vi "sbRIO.vi"() -> ()   [LabVIEW 2012]
uses:
  <vilib>/Platform/TimedLoop/XDataNode/timing_clust.ctl
  <vilib>/Platform/TimedLoop/XDataNode/nitl_modes.ctl
  <vilib>/Platform/TimedLoop/XDataNode/wakeup.ctl
  <vilib>/FPGAPlugInAG/sbRIO-9642/niLvFpga_Open_sbRIO-9642.vi
  <vilib>/rvi/interface/common/dynamic/niFpgaDynamicAddResources.vi
  <vilib>/Utility/error.llb/Error Cluster From Error Code.vi
  <vilib>/rvi/errors/niLvFpgaAdjustHostInterfaceError.vi
  <vilib>/FPGAPlugInAG/Dynamic/niLvFpga_Close_Dynamic.vi
  <vilib>/Platform/TimedLoop/XDataNode/XDataNode.xnode
  <vilib>/rvi/interface/nirviOpenFPGA/nirviOpenFPGA.xnode
  FPGA Bitfiles/ReleaseCandidate_FPGATarget_FPGA_LS4xwvBfOfc.lvbitx
  FPGA.vi
  <vilib>/rvi/interface/nirviReadWriteControl/nirviReadWriteControl.xnode
  <vilib>/rvi/interface/nirviCloseFPGA/nirviCloseFPGA.xnode
  NiFpgaLv.dll
  <vilib>/rvi/interface/Simulation/niFpgaSimulationCallBeginRW.vi
  Helper Functions/ProcessorHelperFunctions.lvlib
  <vilib>/Platform/TimedLoop/XDataNode/XDNodeRunTimeDep.lvlib
panel:
  in  "Error Correction Speed":dbl
  out "Wheel Pos/Speed":picture
  out "Simulation Wheel Angles":dbl[](array[numeric])
  in  "Port":u16=2055 min=1025 step=1
  out "RX Data":T1
  in  "stop":bool
  in  "Manual Motor Control":bool=TRUE
  in  "Motor Number":u8
  out "Chassis Temp (C)":dbl
  out "E1":i64
  out "E3":i64
  out "E2":i64
  out "E4":i64
  out "A1":dbl
  out "A3":dbl
  out "A2":dbl
  out "A4":dbl
  out "T1":dbl
  out "T3":dbl
  out "T2":dbl
  out "T4":dbl
  in  "Calibration Mode":bool
  in  "Debug Mode":bool
  out "Wheel Target Angles":dbl[](array[numeric])
  out "Motor Output Values":u16[](array[slide]) scale=0.0..512.0
  in  "Offset1":i64
  in  "Offset3":i64
  in  "Offset2":i64
  in  "Offset4":i64
  # "Manual Motor Control"
  # "Encoder Count Pre Offset"
  # "Override All"
  # "Automatic\n  Control"
  # "Actual Wheel Angles"
  # "Target Wheel Angles"
  # "Wheel Calibration offsets"
  # "Debug"
  # "(ECS models physical \nparamaters of the robot)"
  # "Normal Operation"
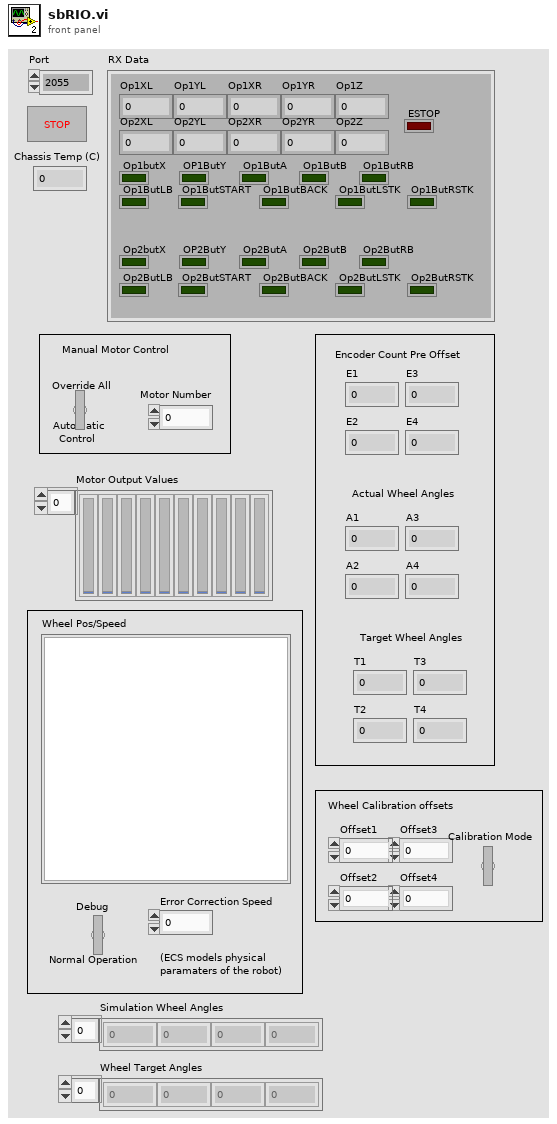
[diagram p1: front panel]
types:
  T1 = cluster{"Op2ButLSTK":bool, "Op2ButRSTK":bool, "Op1ButLSTK":bool, "Op1ButRSTK":bool, "Op1XL":i32, "Op1YL":i32, "Op1XR":i32, "Op1YR":i32, "Op1Z":i32, "Op2XL":i32, "Op2YL":i32, "Op2XR":i32, "Op2YR":i32, "Op2Z":i32, "ESTOP":bool, "Op1butX":bool, "OP1ButY":bool, "Op1ButA":bool, "Op1ButB":bool, "Op1ButRB":bool, "Op1ButLB":bool, "Op2butX":bool, "OP2ButY":bool, "Op2ButA":bool, "Op2ButB":bool, "Op2ButRB":bool, "Op2ButLB":bool, "Op2ButSTART":bool, "Op2ButBACK":bool, "Op1ButSTART":bool, "Op1ButBACK":bool}
  T2 = typedef "XDNodeRunTimeDep.lvlib/timing_clust.ctl" = cluster{"Expected End [f-1]":u64, "Actual End [f-1]":u64, "Finished Late? [f-1]":bool, "Expected End [i-1]":u64, "Actual End [i-1]":u64, "Finished Late? [i-1]":bool, "Expected Start [i]":u64, "Actual Start [i]":u64, "Expected Start [f]":u64, "Actual Start [f]":u64, "Source Name":string, "Structure Name":string, "Period":i64, "Deadline":i64, "Offset":i64, "Start":i64, "Priority":i32, "Timeout":i32, "Mode":T3, "Wakeup Reason":T4, "Error":errorcluster, "Source Type":string, "Secondary Source Type":string, "Global End Time":u64, "Global Start Time":u64, "Frame Duration":u64, "Iteration Duration":u64, "Assigned CPU":i32, "I/O Scan Engine Mode":u32}
  T3 = typedef "XDNodeRunTimeDep.lvlib/nitl_modes.ctl" = enum32{"No Change", "Process missed periods, maintain original phase", "Discard missed periods, maintain original phase", "Process missed periods, ignore original phase", "Discard missed periods, ignore original phase"}
  T4 = typedef "XDNodeRunTimeDep.lvlib/wakeup.ctl" = enum32{"Normal", "Aborted", "Asynchronous wakeup", "Timing source error", "Timed loop error", "Timeout"}
  T5 = cluster{"Target Angles[0]":dbl, "Target Angles[1]":dbl, "Target Angles[2]":dbl, "Target Angles[3]":dbl}
  T6 = cluster{"MotorsOut[0]":u16, "MotorsOut[1]":u16, "MotorsOut[2]":u16, "MotorsOut[3]":u16, "MotorsOut[4]":u16, "MotorsOut[5]":u16, "MotorsOut[6]":u16, "MotorsOut[7]":u16, "MotorsOut[8]":u16, "MotorsOut[9]":u16, "MotorsOut[10]":u16, "MotorsOut[11]":u16}
  T7 = cluster{"[0]":dbl, "[1]":dbl, "[2]":dbl, "[3]":dbl, "[4]":dbl, "[5]":dbl, "[6]":dbl, "[7]":dbl, "[8]":dbl}
  T8 = cluster{"[0]":u16, "[1]":u16, "[2]":u16, "[3]":u16}
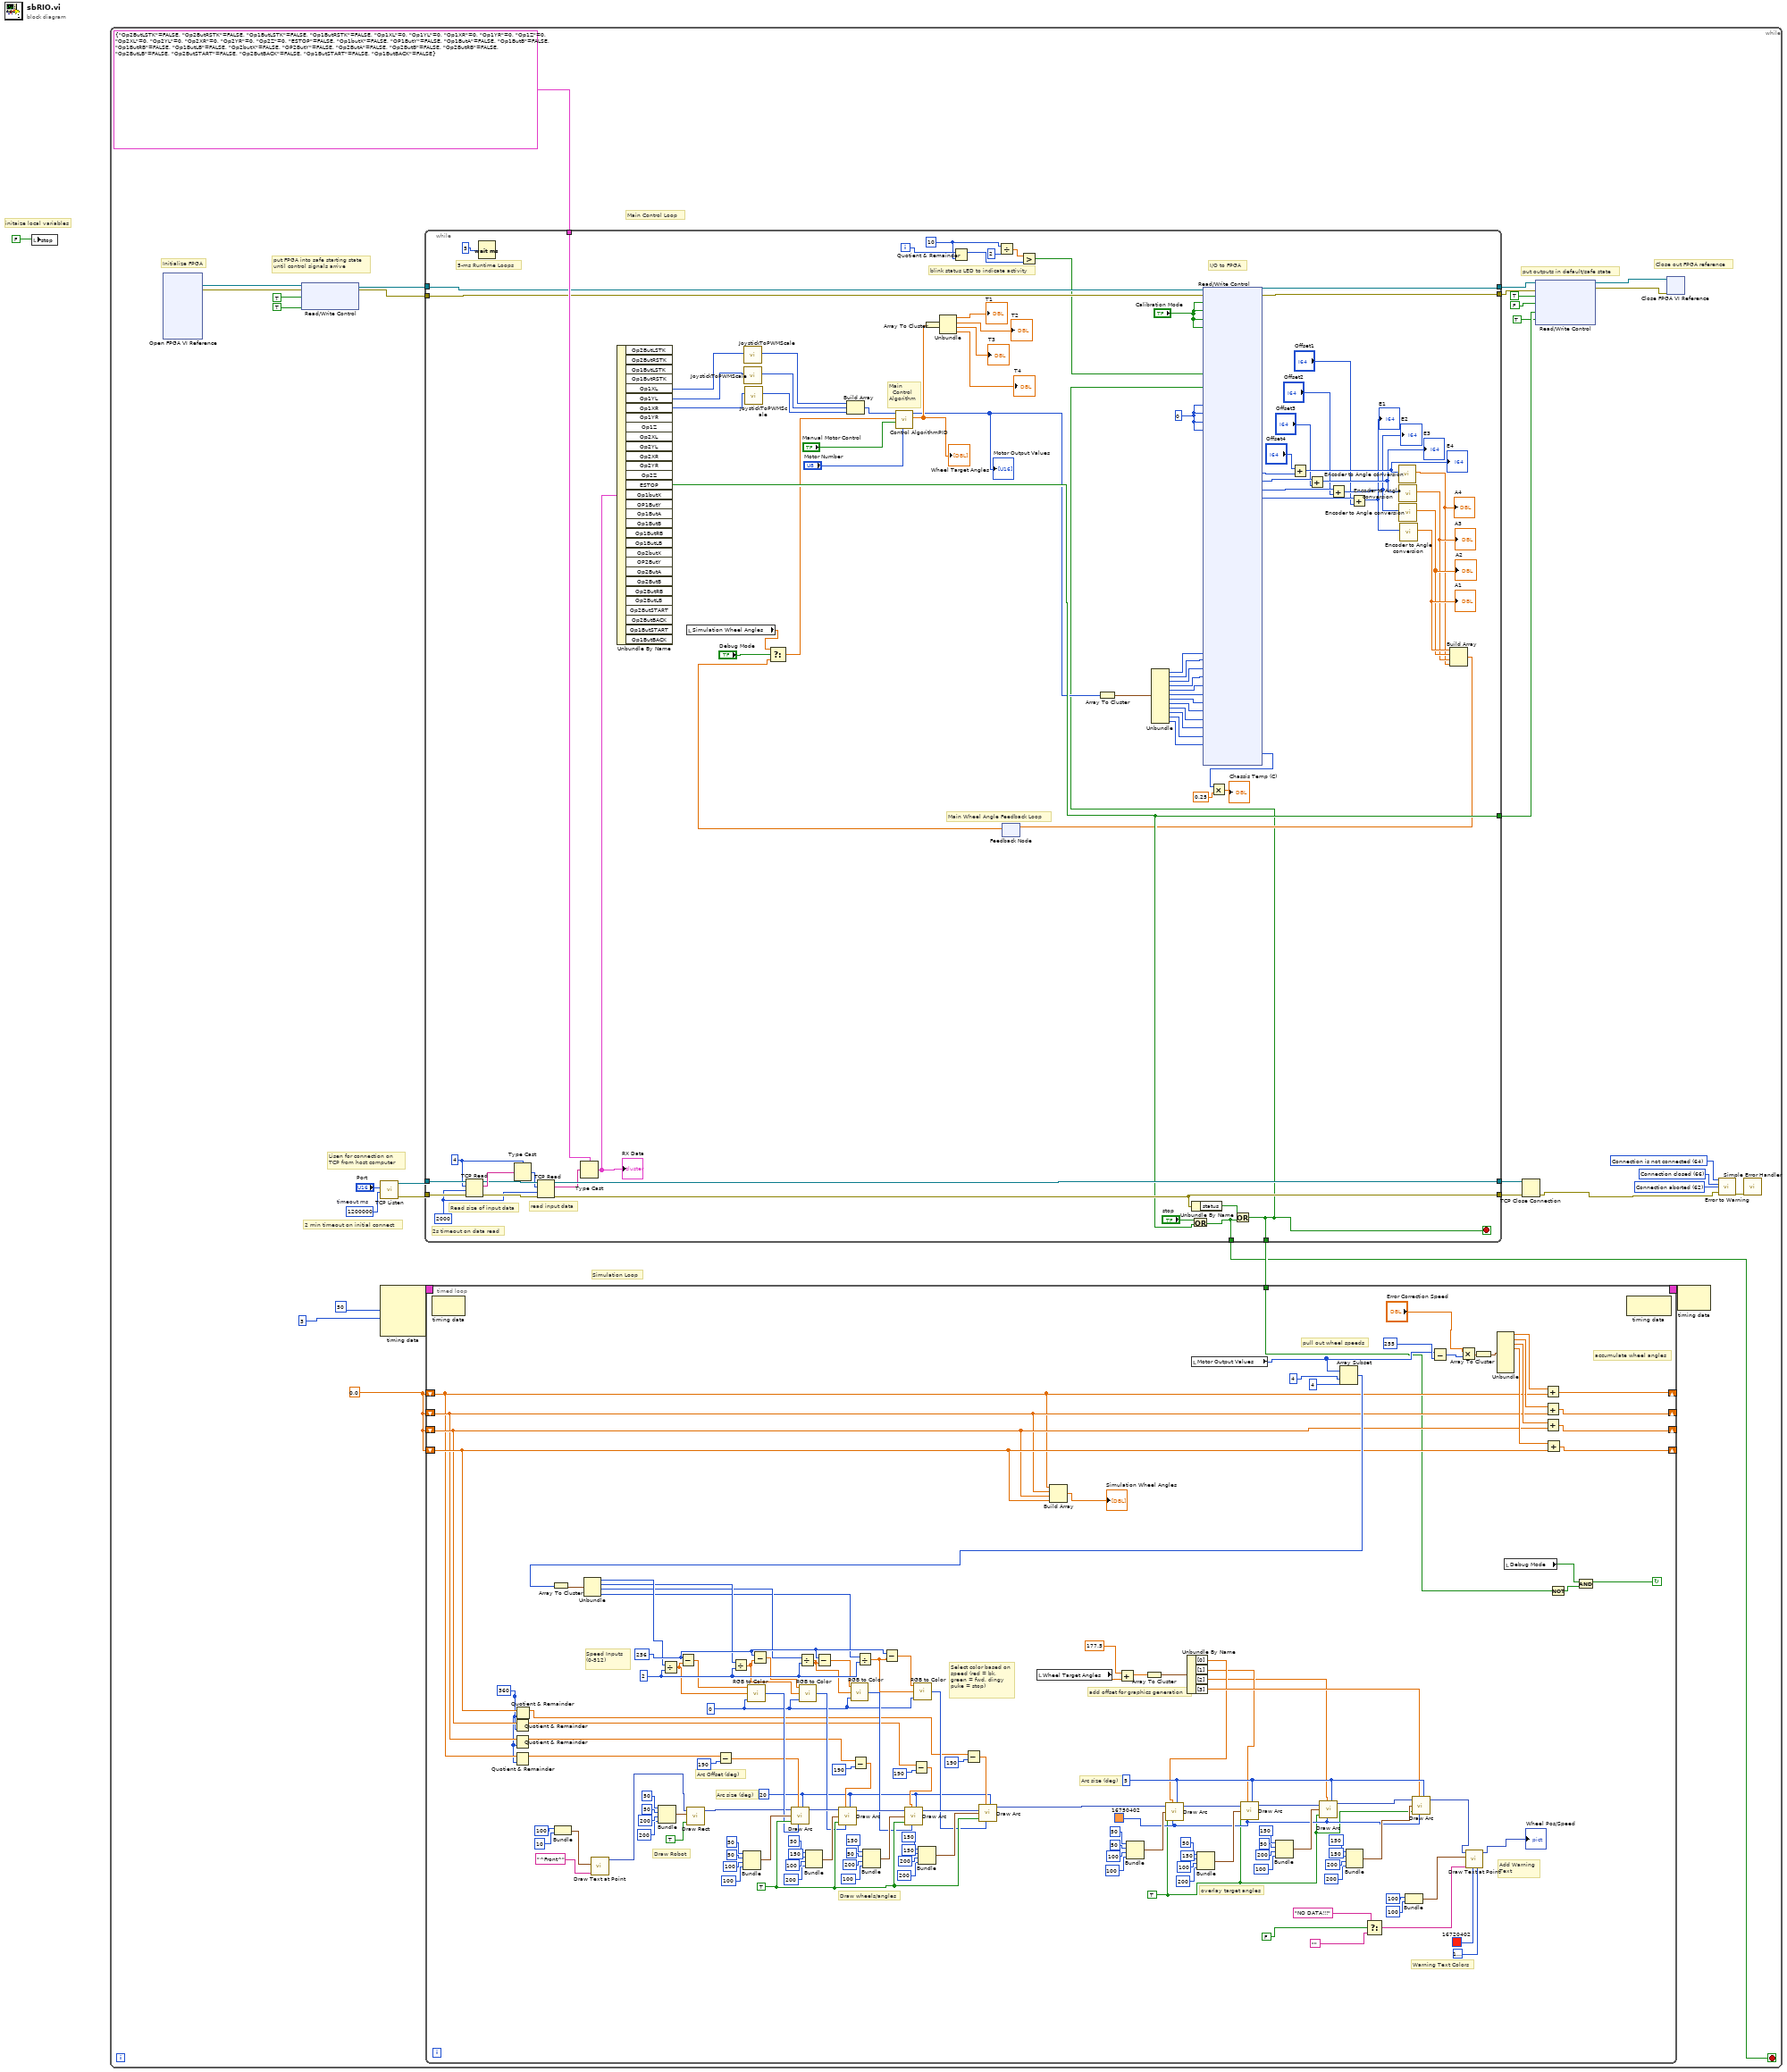
[diagram p0: block diagram]
diagram:
  # "initaize local variables"
  n1 = local write "stop"(FALSE) -> ()
  n2 = while {
    stop <- w2 stop-if-true
    w5 = 0.0
    w25 = 1200000  # timeout ms
    w29 = 62 items=["No Error", "Argument Error", "Memory Full", "Out of Zone", "End of File", "File Already Open", "Generic File IO Error", "File Not Found", "File Permission Error", "Disk Full", "Duplicate Path", "Too Many Files Open", "Not Enabled", "Resource File Not Found", "Cannot Add Resource", "Resource Not Found", "Image Not Found", "Image Memory Error", "Pen Does Not Exist", "Config Bad Type", "Config Token Not Found", "Config Parse Error", "Config Memory Error", "Bad External Code Format", "Bad External Code Offset", "External Code Not Present", "Null Window", "Destroy Window Mixup", "Null Menu", "Print Aborted", "Bad Print Record", "Print Driver Error", "Windows Error During Print", "Memory Error During Print", "Print Dialog Error", "Generic Print Error", "Invalid Device Refnum", "Device Not Found", "Device Parameter Error", "Device Unit Error", "Can't Open Device", "Device Call Aborted", "Generic Error", "Cancelled By User", "Object ID Too Low", "Object ID Too High", "Object Not In Heap", "Unknown Heap", "Bad DefProc ID", "DefProc Not In Table", "Message Out Of Range", "Null Method", "Unknown Message", "Manager Call Not Supported", "Bad address", "Connection In progress", "Connection timed out", "Connection is already in progress", "Network attribute not supported", "Network error", "Address in use", "System out of memory", "Connection aborted", "Connection refused", "Connection is not connected", "Connection is already connected", "Connection closed", "Initialize error (interapplication manager)", "Bad occurrence", "Wait on unbound occurrence handler", "Occurrence queue overflow", "Bad path", "Semaphore not signaled", "Unrecognized type (interapplication manager)"] ("1st Error to Convert")
    w30 = 66 items=["No Error", "Argument Error", "Memory Full", "Out of Zone", "End of File", "File Already Open", "Generic File IO Error", "File Not Found", "File Permission Error", "Disk Full", "Duplicate Path", "Too Many Files Open", "Not Enabled", "Resource File Not Found", "Cannot Add Resource", "Resource Not Found", "Image Not Found", "Image Memory Error", "Pen Does Not Exist", "Config Bad Type", "Config Token Not Found", "Config Parse Error", "Config Memory Error", "Bad External Code Format", "Bad External Code Offset", "External Code Not Present", "Null Window", "Destroy Window Mixup", "Null Menu", "Print Aborted", "Bad Print Record", "Print Driver Error", "Windows Error During Print", "Memory Error During Print", "Print Dialog Error", "Generic Print Error", "Invalid Device Refnum", "Device Not Found", "Device Parameter Error", "Device Unit Error", "Can't Open Device", "Device Call Aborted", "Generic Error", "Cancelled By User", "Object ID Too Low", "Object ID Too High", "Object Not In Heap", "Unknown Heap", "Bad DefProc ID", "DefProc Not In Table", "Message Out Of Range", "Null Method", "Unknown Message", "Manager Call Not Supported", "Bad address", "Connection In progress", "Connection timed out", "Connection is already in progress", "Network attribute not supported", "Network error", "Address in use", "System out of memory", "Connection aborted", "Connection refused", "Connection is not connected", "Connection is already connected", "Connection closed", "Initialize error (interapplication manager)", "Bad occurrence", "Wait on unbound occurrence handler", "Occurrence queue overflow", "Bad path", "Semaphore not signaled", "Unrecognized type (interapplication manager)"] ("1st Error to Convert")
    w31 = 64 items=["No Error", "Argument Error", "Memory Full", "Out of Zone", "End of File", "File Already Open", "Generic File IO Error", "File Not Found", "File Permission Error", "Disk Full", "Duplicate Path", "Too Many Files Open", "Not Enabled", "Resource File Not Found", "Cannot Add Resource", "Resource Not Found", "Image Not Found", "Image Memory Error", "Pen Does Not Exist", "Config Bad Type", "Config Token Not Found", "Config Parse Error", "Config Memory Error", "Bad External Code Format", "Bad External Code Offset", "External Code Not Present", "Null Window", "Destroy Window Mixup", "Null Menu", "Print Aborted", "Bad Print Record", "Print Driver Error", "Windows Error During Print", "Memory Error During Print", "Print Dialog Error", "Generic Print Error", "Invalid Device Refnum", "Device Not Found", "Device Parameter Error", "Device Unit Error", "Can't Open Device", "Device Call Aborted", "Generic Error", "Cancelled By User", "Object ID Too Low", "Object ID Too High", "Object Not In Heap", "Unknown Heap", "Bad DefProc ID", "DefProc Not In Table", "Message Out Of Range", "Null Method", "Unknown Message", "Manager Call Not Supported", "Bad address", "Connection In progress", "Connection timed out", "Connection is already in progress", "Network attribute not supported", "Network error", "Address in use", "System out of memory", "Connection aborted", "Connection refused", "Connection is not connected", "Connection is already connected", "Connection closed", "Initialize error (interapplication manager)", "Bad occurrence", "Wait on unbound occurrence handler", "Occurrence queue overflow", "Bad path", "Semaphore not signaled", "Unrecognized type (interapplication manager)"] ("1st Error to Convert")
    # "Simulation Loop"
    # "Main Control Loop"
    # "put FPGA into safe starting state\nuntil control signals arrive"
    # "put outputs in default/safe state"
    # "Close out FPGA reference"
    # "Initialize FPGA"
    # "2 min timeout on initial connect"
    # "Lisen for connection on \nTCP from host computer"
    n3 = xnode "Open FPGA VI Reference"() -> ("FPGA VI Reference Out"=w16:refnum<k20>, "error out"=w15:errorcluster)  [unwired: 2 in]
    n4 = xnode "Read/Write Control"("FPGA VI Reference In"=w16, "error in"=w15, "Stop All Motors"=TRUE, "Status LED"=TRUE) -> ("FPGA VI Reference Out"=w14:refnum<k20>, "error out"=w13:errorcluster)
    n5 = call <vilib>:"TCP Listen.vi"("timeout ms (wait forever: -1)"=w25, "port"="Port") -> ("error out"=w23:errorcluster, "connection ID"=w24:refnum<k5>)  [unwired: 5 in, 3 out]
    n6 = node-c288(50, 3) -> (w34:T2)  [unwired: 2 in]
    n7 = while {
      tunnel: w23 -> [w261]
      tunnel: w24 -> [w262]
      tunnel: [w263] -> w22
      tunnel: [w258] -> w21
      tunnel: T1 {"Op2ButLSTK"=FALSE, "Op2ButRSTK"=FALSE, "Op1ButLSTK"=FALSE, "Op1ButRSTK"=FALSE, "Op1XL"=0, "Op1YL"=0, "Op1XR"=0, "Op1YR"=0, "Op1Z"=0, "Op2XL"=0, "Op2YL"=0, "Op2XR"=0, "Op2YR"=0, "Op2Z"=0, "ESTOP"=FALSE, "Op1butX"=FALSE, "OP1ButY"=FALSE, "Op1ButA"=FALSE, "Op1ButB"=FALSE, "Op1ButRB"=FALSE, "Op1ButLB"=FALSE, "Op2butX"=FALSE, "OP2ButY"=FALSE, "Op2ButA"=FALSE, "Op2ButB"=FALSE, "Op2ButRB"=FALSE, "Op2ButLB"=FALSE, "Op2ButSTART"=FALSE, "Op2ButBACK"=FALSE, "Op1ButSTART"=FALSE, "Op1ButBACK"=FALSE} -> [w255]
      tunnel: w14 -> [w251]
      tunnel: w13 -> [w250]
      tunnel: [w249] -> w20
      tunnel: [w248] -> w19
      tunnel: [w241] -> w8
      tunnel: [w193] -> w3
      tunnel: [w184] -> w2
      i -> [w247]
      stop <- w193 stop-if-true
      w208 = 0
      w243 = 10
      w254 = 2000
      w259 = 4
      # "Main\n  Control\nAlgorithm"
      # "Main Wheel Angle Feedback Loop"
      # "blink status LED to indicate activity"
      # "I/O to FPGA"
      # "2s timeout on data read"
      # "read input data"
      # "Read size of input data"
      # "5-ms Runtime Loops"
      n8 = TCP Read(connection ID=w262, bytes to read=w259, error in (no error)=w261, 9:w254) -> (connection ID out=w266:refnum<k5>, data out=w267:string, error out=w265:errorcluster)  [unwired: 1 in]
      n9 = Wait (ms)(milliseconds to wait=u32 5) -> ()  [unwired: 1 out]
      n10 = Type Cast(type=w259, x=w267) -> (*(type *) &x=w264:i32)
      n11 = TCP Read(connection ID=w266, bytes to read=w264, error in (no error)=w265, 9:w254) -> (connection ID out=w263:refnum<k5>, data out=w260:string, error out=w258:errorcluster)  [unwired: 1 in]
      n12 = Type Cast(type=w255, x=w260) -> (*(type *) &x=w253:T1)
      "RX Data" <- w253
      n13 = Unbundle By Name(w253) -> ("Op1XL"=w206:i32, "Op1YL"=w205:i32, "Op1XR"=w204:i32, "ESTOP"=w241:bool)  [unwired: 27 out]
      n14 = local read "Simulation Wheel Angles"() -> (w198:dbl[])
      n15 = call "JoystickToPWMScale.vi"("Numeric"=w206) -> ("Numeric 2"=w203:u16)  [unwired: 10 in]
      n16 = call "JoystickToPWMScale.vi"("Numeric"=w205) -> ("Numeric 2"=w202:u16)  [unwired: 10 in]
      n17 = call "JoystickToPWMScale.vi"("Numeric"=w204) -> ("Numeric 2"=w201:u16)  [unwired: 10 in]
      n18 = Build Array(w203, w202, w201) -> (w207:u16[])
      n19 = Quotient & Remainder(x=w247, y=w243) -> (x-y*floor(x/y)=w245:i32)  [unwired: 1 out]
      n20 = Divide(x=w243, y=2) -> (x/y=w244:dbl)
      n21 = feedback #1() -> (w199:dbl[])  [unwired: 1 in]
      n22 = Select(t=w198, s="Debug Mode", f=w199) -> (s? t:f=w196:dbl[])
      n23 = call "Control AlgorithmPID.vi"("Motor to Control"="Motor Number", "Manual Control"="Manual Motor Control", "Angles In"=w196, "JoystickIn"=w207) -> ("Target Angles"=w195:dbl[], "MotorsOut"=w194:u16[])  [unwired: 5 in]
      "Wheel Target Angles" <- w195
      "Motor Output Values" <- w194
      n24 = Array To Cluster(array=w195) -> (cluster=w223:T5)
      n25 = Unbundle(w223) -> ("Target Angles[0]"=→"T1":dbl, "Target Angles[1]"=→"T2":dbl, "Target Angles[2]"=→"T3":dbl, "Target Angles[3]"=→"T4":dbl)
      n26 = Greater?(x=w244, y=w245) -> (0:w242:bool)
      n27 = Array To Cluster(array=w194) -> (cluster=w229:T6)
      n28 = Unbundle(w229) -> ("MotorsOut[0]"=w239:u16, "MotorsOut[1]"=w238:u16, "MotorsOut[2]"=w237:u16, "MotorsOut[3]"=w236:u16, "MotorsOut[4]"=w235:u16, "MotorsOut[5]"=w234:u16, "MotorsOut[6]"=w233:u16, "MotorsOut[7]"=w232:u16, "MotorsOut[8]"=w231:u16, "MotorsOut[9]"=w230:u16, "MotorsOut[10]"=w228:u16, "MotorsOut[11]"=w227:u16)
      n29 = Unbundle By Name(w258) -> ("status"=w257:bool)
      n30 = Or(x="stop", y=w241) -> (x .or. y?=w184:bool)
      n31 = Or(x=w257, y=w184) -> (x .or. y?=w193:bool)
      n32 = xnode "Read/Write Control"("FPGA VI Reference In"=w251, "error in"=w250, "Cal. 4"="Calibration Mode", "Cal. 3"="Calibration Mode", "Cal.2"="Calibration Mode", "Cal.1"="Calibration Mode", "Status LED"=w242, "Stop All Motors"=w193, "Analog 3"=w208, "Analog 1"=w208, "Analog 4"=w208, "Analog 2"=w208, "Motor1"=w239, "Motor2"=w238, "Motor3"=w237, "Motor4"=w236, "Motor5"=w235, "Motor6"=w234, "Motor7"=w233, "Motor8"=w232, "Motor9"=w231, "Motor10"=w230, "Motor11"=w228, "Motor12"=w227) -> ("FPGA VI Reference Out"=w249:refnum<k20>, "error out"=w248:errorcluster, "Encoder4"=w218:i64, "Encoder3"=w217:i64, "Encoder2"=w216:i64, "Encoder1"=w215:i64, "Chasis Temp"=w224:i16)  [unwired: 15 in, 13 out]
      n33 = Multiply(x=w224, y=0.25) -> (x*y=→"Chassis Temp (C)":dbl)
      n34 = Add(x="Offset4", y=w218) -> (x+y=w192:i64)
      "E4" <- w192
      n35 = Add(x=w217, y="Offset3") -> (x+y=w190:i64)
      "E3" <- w190
      n36 = Add(x=w216, y="Offset2") -> (x+y=w189:i64)
      "E2" <- w189
      n37 = Add(x=w215, y="Offset1") -> (x+y=w188:i64)
      "E1" <- w188
      n38 = call "Encoder to Angle conversion.vi"("Input"=w192) -> ("Output"=w211:dbl)  [unwired: 10 in]
      "A4" <- w211
      n39 = call "Encoder to Angle conversion.vi"("Input"=w190) -> ("Output"=w212:dbl)  [unwired: 10 in]
      "A3" <- w212
      n40 = call "Encoder to Angle conversion.vi"("Input"=w189) -> ("Output"=w213:dbl)  [unwired: 10 in]
      "A2" <- w213
      n41 = call "Encoder to Angle conversion.vi"("Input"=w188) -> ("Output"=w214:dbl)  [unwired: 10 in]
      "A1" <- w214
      n42 = Build Array(w214, w213, w212, w211) -> (w210:dbl[])
      n43 = feedback-in #1(w210) -> ()
    }
    n44 = timed-loop {
      timing: w34 -> [_]
      timing-out: [_] -> w33
      shift-right: [w171] -> _
      shift-left: w5 -> [w43]
      shift-right: [w170] -> _
      shift-left: w5 -> [w45]
      shift-right: [w172] -> _
      shift-left: w5 -> [w41]
      shift-right: [w173] -> _
      shift-left: w5 -> [w39]
      tunnel: w3 -> [w35]
      stop <- w37 continue-if-true
      w38 = 360
      w65 = TRUE
      w68 = 5
      w69 = u32 16750402
      w109 = 20
      w111 = 0
      w127 = 2
      w128 = 256
      w140 = TRUE
      # "add offset for graphics generation"
      # "pull out wheel speeds"
      # "Arc size (deg)"
      # "overlay target angles"
      # "Add Warning\nText"
      # "Warning Text Colors"
      # "Arc Offset (deg)"
      # "Arc size (deg)"
      # "Speed Inputs (0-512)"
      # "Draw wheels/angles"
      # "Select color based on speed (red = bk, green = fwd, dingy puke = stop)"
      # "Draw Robot"
      # "accumulate wheel angles"
      n45 = node-c288() -> ()  [unwired: 1 in, 1 out]
      n46 = Quotient & Remainder(x=w43, y=w38) -> (x-y*floor(x/y)=w44:dbl)  [unwired: 1 out]
      n47 = Quotient & Remainder(x=w41, y=w38) -> (x-y*floor(x/y)=w42:dbl)  [unwired: 1 out]
      n48 = Quotient & Remainder(x=w39, y=w38) -> (x-y*floor(x/y)=w40:dbl)  [unwired: 1 out]
      n49 = Quotient & Remainder(x=w45, y=w38) -> (x-y*floor(x/y)=w46:dbl)  [unwired: 1 out]
      n50 = Bundle(100, 10) -> (w104:cluster{i32, i32})  [unwired: 1 in]
      n51 = call <vilib>:"Draw Text at Point.vi"("text"="^Front^", "origin"=w104) -> ("new picture"=w108:picture)  [unwired: 8 in, 1 out]
      n52 = Bundle(50, 50, 200, 200) -> (w131:cluster{i32, i32, i32, i32})  [unwired: 1 in]
      n53 = call <vilib>:"Draw Rect.vi"("picture"=w108, "rect"=w131, "fill?(F)"=TRUE) -> ("new picture"=w129:picture)  [unwired: 6 in]
      n54 = Subtract(x=w40, y=190) -> (x-y=w117:dbl)
      n55 = Bundle(50, 50, 100, 100) -> (w157:cluster{i32, i32, i32, i32})  [unwired: 1 in]
      n56 = Bundle(50, 150, 100, 200) -> (w143:cluster{i32, i32, i32, i32})  [unwired: 1 in]
      n57 = Subtract(x=w42, y=190) -> (x-y=w113:dbl)
      n58 = Bundle(150, 50, 200, 100) -> (w142:cluster{i32, i32, i32, i32})  [unwired: 1 in]
      n59 = Subtract(x=w44, y=190) -> (x-y=w112:dbl)
      n60 = Bundle(150, 150, 200, 200) -> (w141:cluster{i32, i32, i32, i32})  [unwired: 1 in]
      n61 = Subtract(x=w46, y=190) -> (x-y=w110:dbl)
      n62 = local read "Wheel Target Angles"() -> (w54:dbl[])
      n63 = Build Array(w39, w41, w43, w45) -> (→"Simulation Wheel Angles":dbl[])
      n64 = Add(x=177.5, y=w54) -> (x+y=w51:dbl[])
      n65 = Bundle(50, 50, 100, 100) -> (w87:cluster{i32, i32, i32, i32})  [unwired: 1 in]
      n66 = Array To Cluster(array=w51) -> (cluster=w67:T7)
      n67 = Unbundle By Name(w67) -> ("[0]"=w49:dbl, "[1]"=w48:dbl, "[2]"=w47:dbl, "[3]"=w66:dbl)
      n68 = local read "Motor Output Values"() -> (w55:u16[])
      n69 = Bundle(50, 150, 100, 200) -> (w81:cluster{i32, i32, i32, i32})  [unwired: 1 in]
      n70 = Bundle(150, 50, 200, 100) -> (w76:cluster{i32, i32, i32, i32})  [unwired: 1 in]
      n71 = Array Subset(array=w55, index=4, length=4) -> (w60:u16[])
      n72 = Array To Cluster(array=w60) -> (cluster=w61:T8)
      n73 = Unbundle(w61) -> ("[0]"=w59:u16, "[1]"=w58:u16, "[2]"=w57:u16, "[3]"=w56:u16)
      n74 = Divide(x=w59, y=w127) -> (x/y=w126:dbl)
      n75 = Subtract(x=w128, y=w126) -> (x-y=w123:dbl)
      n76 = Divide(x=w58, y=w127) -> (x/y=w125:dbl)
      n77 = call <vilib>:"RGB to Color.vi"("B"=w111, "G"=w126, "R"=w123) -> ("Color"=w139:u32)
      n78 = Subtract(x=w128, y=w125) -> (x-y=w122:dbl)
      n79 = call <vilib>:"Draw Arc.vi"("picture"=w129, "start angle[degrees]"=w117, "rect"=w157, "fill?(F)"=w140, "color(black)"=w139, "arc size[degrees]"=w109) -> ("new picture"=w163:picture)  [unwired: 3 in]
      n80 = Divide(x=w57, y=w127) -> (x/y=w121:dbl)
      n81 = call <vilib>:"RGB to Color.vi"("B"=w111, "G"=w125, "R"=w122) -> ("Color"=w138:u32)
      n82 = Subtract(x=w128, y=w121) -> (x-y=w120:dbl)
      n83 = call <vilib>:"Draw Arc.vi"("picture"=w163, "start angle[degrees]"=w113, "rect"=w143, "fill?(F)"=w140, "color(black)"=w138, "arc size[degrees]"=w109) -> ("new picture"=w162:picture)  [unwired: 3 in]
      n84 = call <vilib>:"RGB to Color.vi"("B"=w111, "G"=w121, "R"=w120) -> ("Color"=w137:u32)
      n85 = Divide(x=w56, y=w127) -> (x/y=w124:dbl)
      n86 = Subtract(x=w128, y=w124) -> (x-y=w119:dbl)
      n87 = call <vilib>:"Draw Arc.vi"("picture"=w162, "start angle[degrees]"=w112, "rect"=w142, "fill?(F)"=w140, "color(black)"=w137, "arc size[degrees]"=w109) -> ("new picture"=w161:picture)  [unwired: 3 in]
      n88 = call <vilib>:"RGB to Color.vi"("B"=w111, "G"=w124, "R"=w119) -> ("Color"=w136:u32)
      n89 = call <vilib>:"Draw Arc.vi"("picture"=w161, "start angle[degrees]"=w110, "rect"=w141, "fill?(F)"=w140, "color(black)"=w136, "arc size[degrees]"=w109) -> ("new picture"=w93:picture)  [unwired: 3 in]
      n90 = call <vilib>:"Draw Arc.vi"("picture"=w93, "start angle[degrees]"=w49, "rect"=w87, "fill?(F)"=w65, "color(black)"=w69, "arc size[degrees]"=w68) -> ("new picture"=w92:picture)  [unwired: 3 in]
      n91 = call <vilib>:"Draw Arc.vi"("picture"=w92, "start angle[degrees]"=w48, "rect"=w81, "fill?(F)"=w65, "color(black)"=w69, "arc size[degrees]"=w68) -> ("new picture"=w75:picture)  [unwired: 3 in]
      n92 = call <vilib>:"Draw Arc.vi"("picture"=w75, "start angle[degrees]"=w47, "rect"=w76, "fill?(F)"=w65, "color(black)"=w69, "arc size[degrees]"=w68) -> ("new picture"=w91:picture)  [unwired: 3 in]
      n93 = Bundle(150, 150, 200, 200) -> (w70:cluster{i32, i32, i32, i32})  [unwired: 1 in]
      n94 = Select(t="NO DATA!!!", s=FALSE, f="") -> (s? t:f=w97:string)
      n95 = Bundle(100, 100) -> (w100:cluster{i32, i32})  [unwired: 1 in]
      n96 = call <vilib>:"Draw Arc.vi"("picture"=w91, "start angle[degrees]"=w66, "rect"=w70, "fill?(F)"=w65, "color(black)"=w69, "arc size[degrees]"=w68) -> ("new picture"=w94:picture)  [unwired: 3 in]
      n97 = Subtract(x=w55, y=255) -> (x-y=w175:i32[])
      n98 = Multiply(x="Error Correction Speed", y=w175) -> (x*y=w169:dbl[])
      n99 = call <vilib>:"Draw Text at Point.vi"("BG color(transparent)"=u32 16777216, "text color(black)"=u32 16720402, "text"=w97, "origin"=w100, "picture"=w94) -> ("new picture"=→"Wheel Pos/Speed":picture)  [unwired: 5 in, 1 out]
      n100 = Array To Cluster(array=w169) -> (cluster=w174:T7)
      n101 = Unbundle(w174) -> ("[0]"=w167:dbl, "[1]"=w166:dbl, "[2]"=w165:dbl, "[3]"=w164:dbl)  [unwired: 5 out]
      n102 = local read "Debug Mode"() -> (w52:bool)
      n103 = Add(x=w167, y=w39) -> (x+y=w173:dbl)
      n104 = Add(x=w166, y=w41) -> (x+y=w172:dbl)
      n105 = Add(x=w165, y=w43) -> (x+y=w171:dbl)
      n106 = Add(x=w164, y=w45) -> (x+y=w170:dbl)
      n107 = Not(x=w35) -> (.not. x?=w36:bool)
      n108 = And(x=w52, y=w36) -> (x .and. y?=w37:bool)
      n109 = node-c288() -> ()  [unwired: 1 in, 1 out]
    }
    n110 = TCP Close Connection(connection ID=w22, error in (no error)=w21) -> (error out=w27:errorcluster)  [unwired: 1 in, 1 out]
    n111 = xnode "Read/Write Control"("FPGA VI Reference In"=w20, "error in"=w19, "Stop All Motors"=TRUE, "Status LED"=FALSE, "Emergency Stop"=w8, "Halt Execution"=TRUE) -> ("FPGA VI Reference Out"=w18:refnum<k20>, "error out"=w11:errorcluster)
    n112 = xnode "Close FPGA VI Reference"("FPGA VI Reference In"=w18, "error in"=w11) -> ()  [unwired: 1 out]
    n113 = node-c288(w33) -> ()  [unwired: 1 out]
    n114 = call <vilib>:"Error to Warning.vi"("1st Error to Convert"=w31, "2nd Error to Convert"=w30, "3rd Error to Convert"=w29, "error in"=w27) -> ("warning out"=w32:errorcluster)  [unwired: 11 in]
    n115 = call <vilib>:"Simple Error Handler.vi"("error in (no error)"=w32) -> ()  [unwired: 4 in, 5 out]
  }
